vi "Reaction Wheel Controller.vi"(11 "Cluster":cluster{}) -> ()   [LabVIEW 2021]
panel:
  out "Error":dbl
  out "PID output":dbl
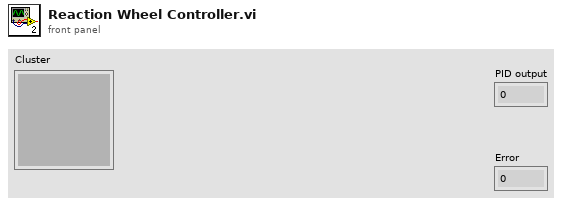
[diagram p1: front panel]
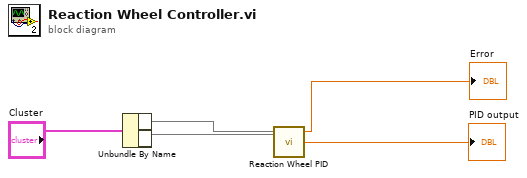
[diagram p0: block diagram]
diagram:
  n1 = Unbundle By Name("Cluster") -> (w1, w4)
  n2 = call "Reaction Wheel PID.vi"("Roll"=w4, "Roll reference"=w1) -> ("PID output"=→"PID output":dbl, "Ref. error"=→"Error":dbl)  [unwired: 2 in]
